vi "Toggle Debug Mode.vi"(8 "error in (no error)":errorcluster) -> (0 "error out":errorcluster)   [LabVIEW 2015, in "Main Controller Actor API.lvclass"]
uses:
  Main Controller Actor API.lvclass
  Re-use Libraries/Minimal Actor Framework/Messaging/Message/Message.lvclass/Message.ctl
  Globals.vi
  Re-use Libraries/Minimal Actor Framework/Messaging/Message/Message.lvclass
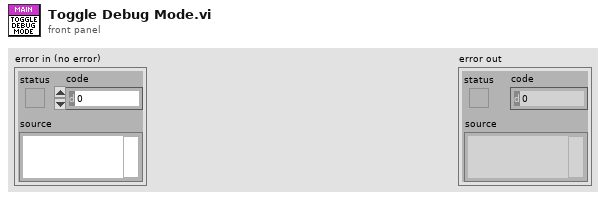
[diagram p1: front panel]
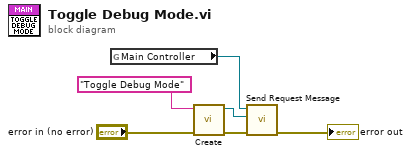
[diagram p0: block diagram]
diagram:
  n1 = global read "Globals.vi" "Main Controller"() -> (w3:refnum<class "Main Controller Actor API.lvclass">)
  n2 = call "Create.vi"("error in (no error)"="error in (no error)", "Name"="Toggle Debug Mode" ("Parameter")) -> ("error out"=w4:errorcluster, "Message out"=w5:refnum<class "Message.lvclass">)  [unwired: 8 in]
  n3 = call-dynamic "Send Request Message.vi"("error in (no error)"=w4, "Message"=w5, "Actor API in"=w3) -> ("error out"=→"error out":errorcluster)  [unwired: 8 in]
